vi "Monitor Data Queue.vi"(6 "Queue Function":T1, 8 "error in (no error)":errorcluster, 10 "Max Queue Size(-1)":i32=-1, 11 "Data From FIFO":T2[](array[typedef])) -> (0 "error out":errorcluster, 1 "Queue overflow?":bool, 2 "Last Queue Element":T2, 3 "Queue Elements":T2[](array[typedef]))   [LabVIEW 2016]
uses:
  Typedefs/Monitor Data Element.ctl
  Typedefs/Monitor Data Operation.ctl
panel:
  out "# elements in queue":i32
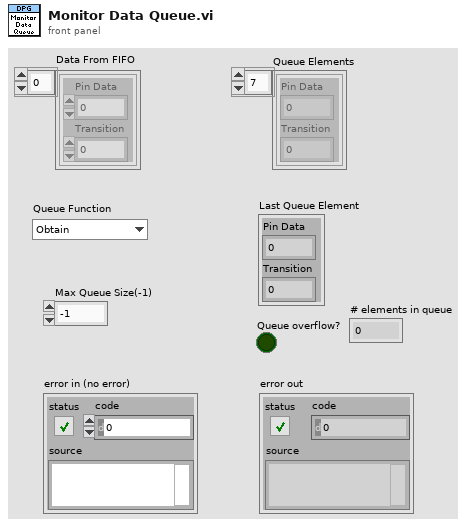
[diagram p1: front panel]
types:
  T1 = typedef "Monitor Data Operation.ctl" = enum16{"Obtain", "Enqueue", "Read Elements", "Flush", "Release", "Read Last Element"}
  T2 = typedef "Monitor Data Element.ctl" = cluster{"Pin Data":u32, "Transition ":u32}
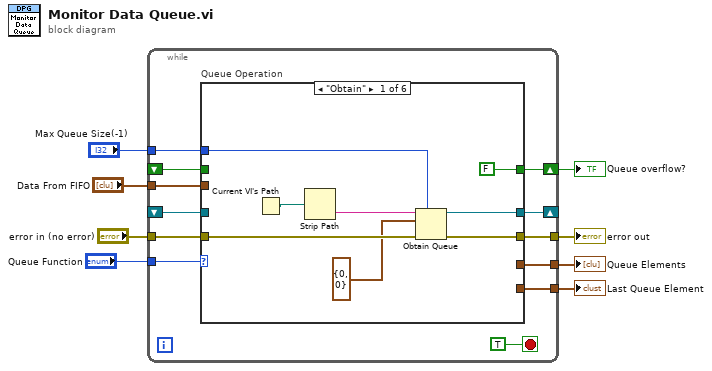
[diagram p0: block diagram]
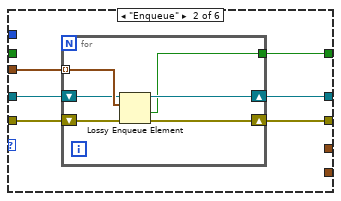
[diagram p2: hidden frame]
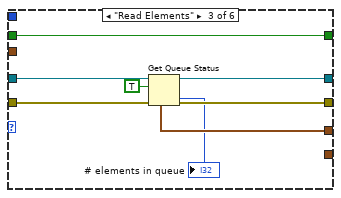
[diagram p3: hidden frame]
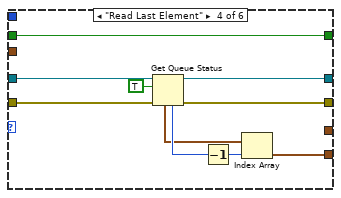
[diagram p4: hidden frame]
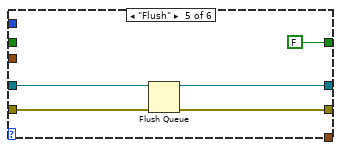
[diagram p5: hidden frame]
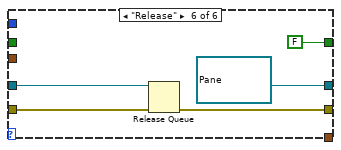
[diagram p6: hidden frame]
diagram:
  n1 = while {
    tunnel: "Queue Function" -> [w19]
    tunnel: "error in (no error)" -> [w17]
    tunnel: [w18] -> w7
    shift-right: [w13] -> _
    shift-left: _ -> [w12]
    tunnel: "Data From FIFO" -> [w16]
    tunnel: [w15] -> w5
    tunnel: [w14] -> w4
    shift-right: [w11] -> w3
    shift-left: _ -> [w10]
    tunnel: "Max Queue Size(-1)" -> [w9]
    stop <- TRUE stop-if-true
    n2 = case "Queue Operation" shown="\"Obtain\"" w19 {
      tunnel: [w27 w33 w47 w57 w62 w67] -> w18
      tunnel: w17 -> [w28 w34 w48 w58 w63 w68]
      tunnel: w16 -> [_ w32 _ _ _ _]
      tunnel: [_ _ w46 _ _ _] -> w15
      tunnel: [_ _ _ w53 _ _] -> w14
      tunnel: [w25 w30 w44 w50 w60 refnum<queue> refnum ("queue out")] -> w13
      tunnel: w12 -> [_ w31 w43 w51 w61 w66]
      tunnel: [FALSE ("overflow?") w29 w42 w49 FALSE ("overflow?") FALSE ("overflow?")] -> w11
      tunnel: w10 -> [_ _ w42 w49 _ _]
      tunnel: w9 -> [w21 _ _ _ _ _]
      frame "Obtain" {
        n3 = Current VI's Path() -> (path=w23:path)
        n4 = Strip Path(path=w23) -> (name=w22:string)  [unwired: 1 out]
        n5 = Obtain Queue(max queue size (-1, unlimited)=w21, name (unnamed)=w22, element data type=T2 {"Pin Data"=0, "Transition "=0}, error in (no error)=w28) -> (queue out=w25:refnum<queue>, error out=w27:errorcluster)  [unwired: 1 in, 1 out]
      }
      frame "Enqueue" {
        n6 = for {
          shift-right: [w37] -> w30
          shift-left: w31 -> [w38]
          tunnel: w32 -> [w39] mode=indexing
          shift-right: [w36] -> w33
          shift-left: w34 -> [w40]
          tunnel: [w35] -> w29
          n7 = Lossy Enqueue Element(queue=w38, element=w39, error in (no error)=w40) -> (queue out=w37:refnum<queue>, overflow?=w35:bool, error out=w36:errorcluster)  [unwired: 1 out]
        }
      }
      frame "Read Elements" {
        n8 = Get Queue Status(queue=w43, return elements? (F)=TRUE, error in (no error)=w48) -> (queue out=w44:refnum<queue>, error out=w47:errorcluster, # elements in queue=→"# elements in queue":i32, elements=w46:T2[])  [unwired: 4 out]
      }
      frame "Read Last Element" {
        n9 = Get Queue Status(queue=w51, return elements? (F)=TRUE, error in (no error)=w58) -> (queue out=w50:refnum<queue>, error out=w57:errorcluster, # elements in queue=w56:i32, elements=w55:T2[])  [unwired: 4 out]
        n10 = Decrement(x=w56) -> (x-1=w54:i32)
        n11 = Index Array(array=w55, index=w54) -> (element=w53:T2)
      }
      frame "Flush" {
        n12 = Flush Queue(queue=w61, error in (no error)=w63) -> (queue out=w60:refnum<queue>, error out=w62:errorcluster)  [unwired: 1 out]
      }
      frame "Release" {
        n13 = Release Queue(queue=w66, error in (no error)=w68) -> (error out=w67:errorcluster)  [unwired: 1 in, 2 out]
      }
    }
  }
  "error out" <- w7
  "Queue Elements" <- w5
  "Last Queue Element" <- w4
  "Queue overflow?" <- w3
